vi "mp.vi"(6 "DLLPath":path, 7 "Draw":enum16{"I(Ewe)", "Ewe(t)", "I(t)", "Test"}(ring)=enum."Ewe(t)", 8 "error in (no error)":errorcluster, 9 "MP Parameters":T3={"tb"=5e-05, "Scans"=[{"Value_step"=0.1, "Duration_step"=0.1, " vs_initial "=FALSE, "Record_every_dT"=0.01, "Record_every_dM"=0.01, "Mode_step"=0}, {"Value_step"=-0.2, "Duration_step"=0.1, " vs_initial "=FALSE, "Record_every_dT"=0.01, "Record_every_dM"=0.01, "Mode_step"=0}, {"Value_step"=0.0, "Duration_step"=0.1, " vs_initial "=FALSE, "Record_every_dT"=0.01, "Record_every_dM"=0.01, "Mode_step"=0}], "I_Range"=12, "Bandwidth"=5, "N_Cycles"=0, "Record_every_rc"=2, "ce"=0, "em"=1, "Step_number"=0} {"Step_number" min=0 max=1000000; "ce" items=["Standard", "CE to ground"]; "N_Cycles" min=0 max=1000000; "Bandwidth" items=["1"=1, "2"=2, "3"=3, "4"=4, "5"=5, "6"=6, "7"=7, "8"=8, "9"=9]; "I_Range" items=["1pA", "1nA", "10nA", "100nA", "1µA", "10µA", "100µA", "1mA", "10mA", "100mA", "1A", "Booster", "Auto"]; "tb" min=5e-05 max=1 format="%^_3e"; "Scans"."Mode_step" min=0 max=1000000; "Scans"."Record_every_dM" format="%^_3e"; "Scans"."Record_every_dT" format="%^_3e"; "Scans"."Duration_step" min=1e-05 max=10 format="%^_3e"; "Scans"."Value_step" format="%^_3e"}, 10 "Channel":u8(ring) items=["1", "2", "3", "4", "5", "6", "7", "8", "9", "10", "11", "12", "13", "14", "15", "16"], 11 "IP adress":string="192.109.209.229") -> (0 "error out":errorcluster, 1 "XY Graph":cluster{"Data 101":sgl[], "Data 101":sgl[]}(graph)={"Data 101"=[8e-05, 0.1006, 0.20111999, 0.30164, 0.40219998, 0.50272, 0.60324, 0.70375997, 0.80428, 0.90484, 1.002, 1.10252, 1.20304, 1.30356, 1.40412, 1.50464, 1.60516, 1.70568, 1.8061999, 1.90676, 2.0072799, 2.1078, 2.20832, 2.3088799, 2.4094, 2.50992, 2.61044, 2.711, 2.8115199, 2.91204, 3.01256, 3.1131198, 3.21364, 3.3141599, 3.41468, 3.5152, 3.6157598, 3.71628, 3.8167999, 3.91732, 4.00108, 4.1015997, 4.20212, 4.30264, 4.4031997, 4.50372, 4.60424, 4.70476, 4.8052797, 4.90584, 5.00636, 5.1068797, 5.2074, 5.30796, 5.4084797, 5.509, 5.60952, 5.7100797, 5.8106, 5.91112], "Data 101"=[4.2835555e-07, 2.1494968e-06, 4.146294e-06, 6.138965e-06, 8.133681e-06, 1.0123058e-05, 1.2087297e-05, 1.4083101e-05, 1.6065378e-05, 1.80591e-05, 1.9984154e-05, 1.7937375e-05, 1.595267e-05, 1.3964497e-05, 1.197563e-05, 9.982255e-06, 7.9902675e-06, 6.0027883e-06, 3.9787647e-06, 1.9855738e-06, -3.2822256e-09, -1.9828094e-06, -3.9722895e-06, -5.9632257e-06, -7.95541e-06, -9.9489125e-06, -1.1902557e-05, -1.389385e-05, -1.5878555e-05, -1.7874703e-05, -1.9867039e-05, -2.1852784e-05, -2.3842693e-05, -2.583641e-05, -2.7823196e-05, -2.9813451e-05, -3.180405e-05, -3.3791526e-05, -3.5780395e-05, -3.777169e-05, -3.9435956e-05, -3.7391255e-05, -3.539476e-05, -3.3405893e-05, -3.1415642e-05, -2.9424347e-05, -2.7433402e-05, -2.5453895e-05, -2.3455323e-05, -2.1465068e-05, -1.9473428e-05, -1.7484906e-05, -1.5494306e-05, -1.3505094e-05, -1.1516228e-05, -9.523894e-06, -7.5357216e-06, -5.542347e-06, -3.5301439e-06, -1.543508e-06]}, 2 "test_output":T1, 3 "Exit 2":bool=TRUE)   [LabVIEW 2022 SP3]
doc: "The VSCAN ( Potentiodynamic Technique) consists of scanning linearly the potential of a stationary working electrode with different scan rates.\nIn general, in this VI, the first thing to do is to start by establishing the connection with the instrument defined by its IP adress, then load the firmware in the channel selected, get the information on the plugged channels, load protocol on a channel, start/stop the protocol, retreive data and draw the graph."
uses:
  Library/EClib Functions/MPParameters.ctl
  Library/EClib Functions/Parameters.ctl
  Library/EClib Functions/EClib functions.lvlib
panel:
  out "mp_data":T2
  in  "Display Parameters?":bool caption="Display Parameters"
  out "DllPath":path caption="DLL Path"
  out "LibVersion":string caption="DLL Version"
  out "Device Code":i32=12
  out "Number of points":i32=60
  out "Data 124":sgl[][](array[numeric])=[[8e-05, -0.00015008324, 4.2835555e-07, 0.0013634439, 1.0], [0.1006, 0.009902848, 2.1494968e-06, 0.010471455, 1.0], [0.20111999, 0.019955778, 4.146294e-06, 0.02059764, 1.0], [0.30164, 0.030008709, 6.138965e-06, 0.030609425, 1.0], [0.40219998, 0.04006164, 8.133681e-06, 0.04071481, 1.0], [0.50272, 0.050114572, 1.0123058e-05, 0.05077513, 1.0], [0.60324, 0.060167503, 1.2087297e-05, 0.06075918, 1.0], [0.70375997, 0.07022043, 1.4083101e-05, 0.07082297, 1.0], [0.80428, 0.08027337, 1.6065378e-05, 0.080852084, 1.0], [0.90484, 0.090326294, 1.80591e-05, 0.090902, 1.0], [1.002, 0.10004413, 1.9984154e-05, 0.100629516, 1.0], [1.10252, 0.0899912, 1.7937375e-05, 0.09124173, 1.0], [1.20304, 0.07993827, 1.595267e-05, 0.08120915, 1.0], [1.30356, 0.069885336, 1.3964497e-05, 0.0711627, 1.0], [1.40412, 0.059832405, 1.197563e-05, 0.06106771, 1.0], [1.50464, 0.049779475, 9.982255e-06, 0.051007397, 1.0], [1.60516, 0.039726544, 7.9902675e-06, 0.040967878, 1.0], [1.70568, 0.029673612, 6.0027883e-06, 0.030924892, 1.0], [1.8061999, 0.019620681, 3.9787647e-06, 0.020868042, 1.0], [1.90676, 0.009567751, 1.9855738e-06, 0.010804256, 1.0], [2.0072799, -0.00048518094, -3.2822256e-09, 0.0006746042, 1.0], [2.1078, -0.010538111, -1.9828094e-06, -0.009257445, 1.0], [2.20832, -0.020591041, -3.9722895e-06, -0.019307364, 1.0], [2.3088799, -0.030643972, -5.9632257e-06, -0.029412746, 1.0], [2.4094, -0.0406969, -7.95541e-06, -0.039452266, 1.0], [2.50992, -0.050749835, -9.9489125e-06, -0.049533386, 1.0], [2.61044, -0.060802765, -1.1902557e-05, -0.059479296, 1.0], [2.711, -0.07085569, -1.389385e-05, -0.06955695, 1.0], [2.8115199, -0.08090863, -1.5878555e-05, -0.07963461, 1.0], [2.91204, -0.09096155, -1.7874703e-05, -0.08969492, 1.0], [3.01256, -0.10101449, -1.9867039e-05, -0.09973444, 1.0], [3.1131198, -0.111067414, -2.1852784e-05, -0.1098225, 1.0], [3.21364, -0.12112035, -2.3842693e-05, -0.119851604, 1.0], [3.3141599, -0.13117327, -2.583641e-05, -0.12988071, 1.0], [3.41468, -0.1412262, -2.7823196e-05, -0.13995838, 1.0], [3.5152, -0.15127914, -2.9813451e-05, -0.15000136, 1.0], [3.6157598, -0.16133207, -3.180405e-05, -0.16006514, 1.0], [3.71628, -0.17138499, -3.3791526e-05, -0.1701324, 1.0], [3.8167999, -0.18143792, -3.5780395e-05, -0.18019964, 1.0], [3.91732, -0.19149086, -3.777169e-05, -0.19023915, 1.0], [4.00108, -0.1998683, -3.9435956e-05, -0.19861813, 1.0], [4.1015997, -0.18981537, -3.7391255e-05, -0.1892373, 1.0], [4.20212, -0.17976244, -3.539476e-05, -0.17914924, 1.0], [4.30264, -0.1697095, -3.3405893e-05, -0.16911319, 1.0], [4.4031997, -0.15965658, -3.1415642e-05, -0.15908061, 1.0], [4.50372, -0.14960365, -2.9424347e-05, -0.14899254, 1.0], [4.60424, -0.13955072, -2.7433402e-05, -0.13895303, 1.0], [4.70476, -0.12949778, -2.5453895e-05, -0.12891698, 1.0], [4.8052797, -0.119444855, -2.3455323e-05, -0.11883587, 1.0], [4.90584, -0.10939193, -2.1465068e-05, -0.10876862, 1.0], [5.00636, -0.09933899, -1.9473428e-05, -0.098690964, 1.0], [5.1068797, -0.08928607, -1.7484906e-05, -0.088686116, 1.0], [5.2074, -0.07923313, -1.5494306e-05, -0.07859806, 1.0], [5.30796, -0.069180205, -1.3505094e-05, -0.06854121, 1.0], [5.4084797, -0.059127275, -1.1516228e-05, -0.05848783, 1.0], [5.509, -0.049074344, -9.523894e-06, -0.048455246, 1.0], [5.60952, -0.039021414, -7.5357216e-06, -0.038367193, 1.0], [5.7100797, -0.028968483, -5.542347e-06, -0.028327677, 1.0], [5.8106, -0.018915553, -3.5301439e-06, -0.018236158, 1.0], [5.91112, -0.008862623, -1.543508e-06, -0.008182773, 1.0]] format="%.2f"
  in  "stop":bool
  in  "Exit":bool
  in  "Start":bool
  # "Instructions:\nBefore running the VI you must type a valid IP adress that corresponds to the instrument.Then press the Run button to execute this VI.\nWhile this VI is running, choose the available channel, enter the MP parameters or keep the default values, then press the button start to begin the experience.\nChoose the waveform to draw (Ewe(t) or I(t) or I(Ewe) or Ec(t). You can stop the measure if you press the stop button and exit the execution if you press the exit button."
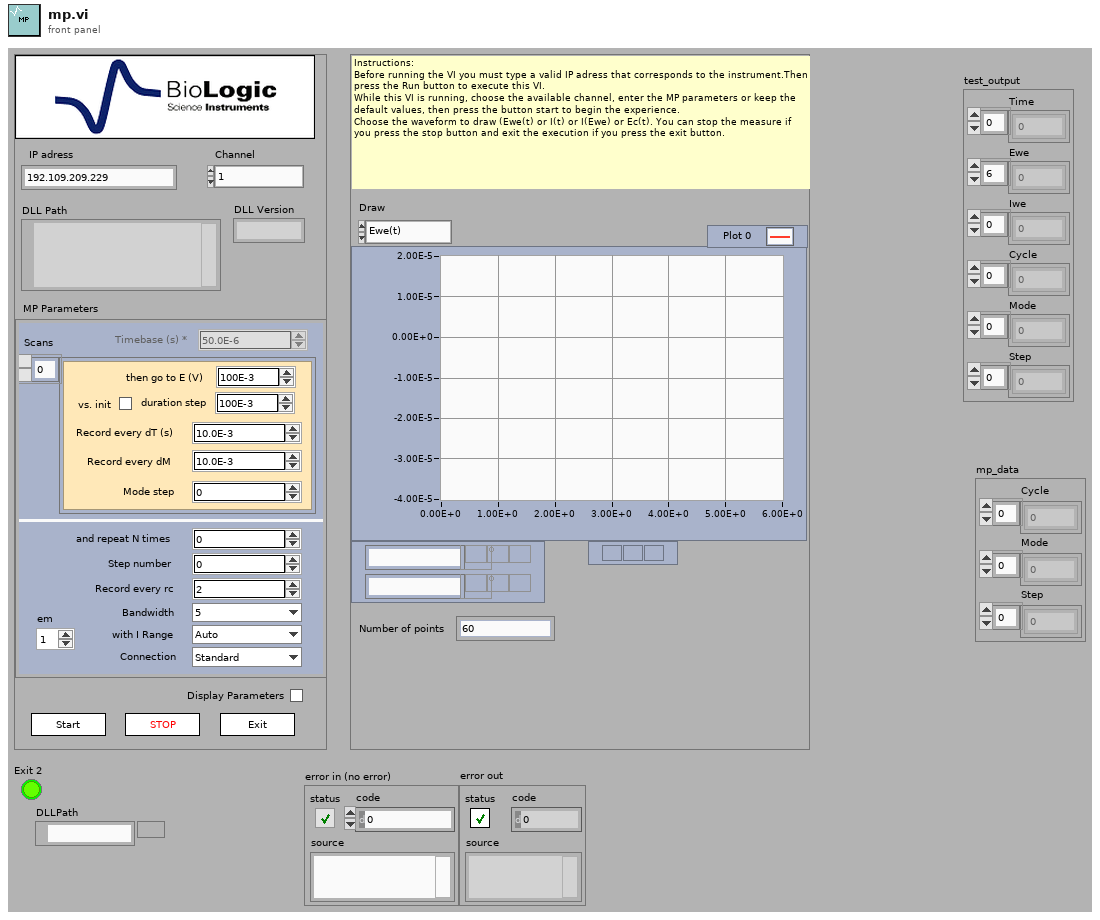
[diagram p1: front panel]
types:
  T1 = cluster{"Time":sgl[], "Ewe":sgl[], "Iwe":sgl[], "Cycle":u32[], "Mode":u32[], "Step":u32[]}
  T2 = cluster{"Cycle":u32[], "Mode":u32[], "Step":u32[]}
  T3 = typedef "EClib functions.lvlib/MPParameters.ctl" = cluster{"tb":sgl, "Scans":cluster{"Value_step":sgl, "Duration_step":sgl, " vs_initial ":bool, "Record_every_dT":sgl, "Record_every_dM":sgl, "Mode_step":i32}[], "I_Range":u16, "Bandwidth":u16, "N_Cycles":i32, "Record_every_rc":i32, "ce":u16, "em":u16, "Step_number":i32}
  T4 = cluster{"LibVersion":string, "StringLength":u32, "DllPath":path}
  T5 = cluster{"Channel":i32, "BoardVersion":i32, "BoardSerialCode":i32, "FirmwareCode":i32, "FirmwareVersion":i32, "XilinxVersion":i32, "AmpCode":i32, "NbAmp":i32, "LcBoard":i32, "Zboard":i32, "MuxBoard":i32, "GPRAboard":i32, "MemSize":i32, "MemFilled":i32, "state":i32, "MaxIRange":i32, "MinIRange":i32, "MaxBandwidth":i32, "NbOfTechniques":i32}
  T6 = typedef "EClib functions.lvlib/Parameters.ctl" = enum16{"CA", "CASG", "CP", "GEIS", "ISCAN", "OCV", "PEIS", "SCCX", "SGEIS", "SPEIS", "VSCAN", "MP"}
  T7 = typedef "EClib functions.lvlib/TechniqueParameters.ctl" = cluster{"String Label":string, "Type":i32, "Valeur":i32, "Index":i32}
  T8 = cluster{"string before end tag":string, i32, i32, i32}[]
  T9 = cluster{"IRQskipped":i32, "NbRaws":i32, "NbCols":i32, "Technique Index":i32, "TechniqueID":i32, "PrcessIndex":i32, "loop":i32, "StartTime":dbl, "MuxPad":i32}
  T10 = cluster{"State":i32, "MemFilled":i32, "TimeBase":sgl, " Ewe":sgl, " EweRangeMin":sgl, " EweRangeMax":sgl, "Ece":sgl, "EceRangeMin":sgl, "EceRangeMax":sgl, "Eoverflow":i32, "I":sgl, "IRange":i32, "Ioverflow":i32, "ElapsedTime":sgl, "Freq":sgl, "Rcomp":sgl, "Saturation":sgl, "OptErr":i32, "OptPos":i32}
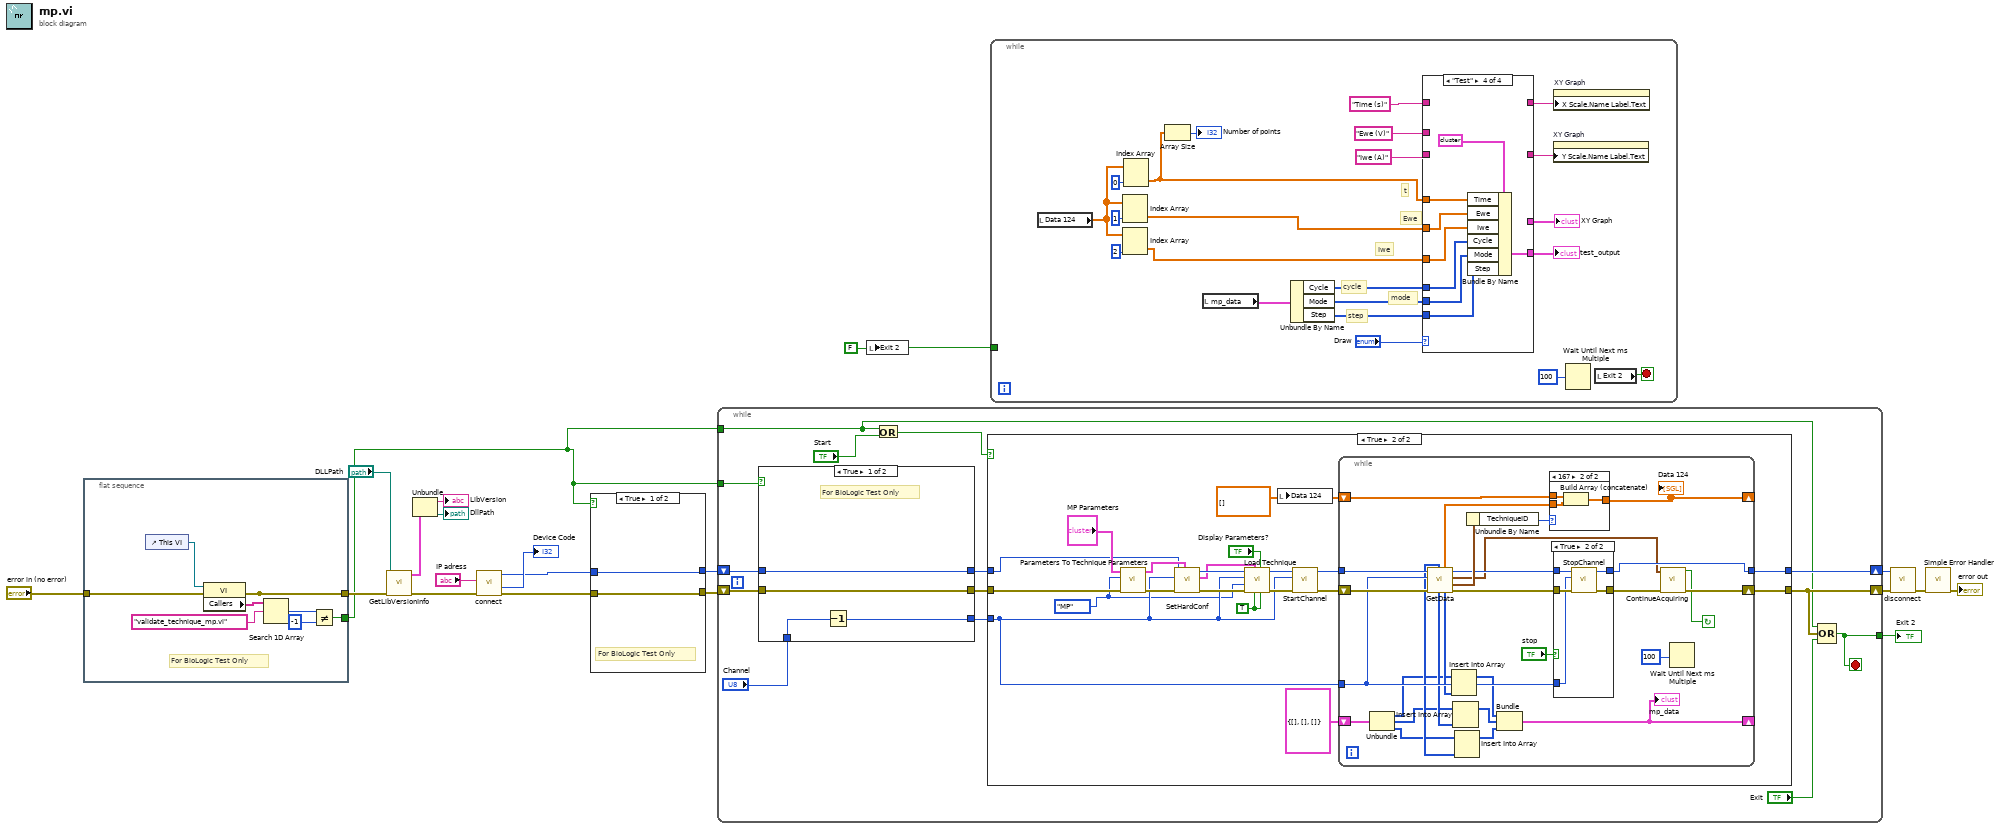
[diagram p0: block diagram]
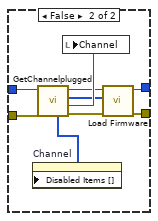
[diagram p2: hidden frame]
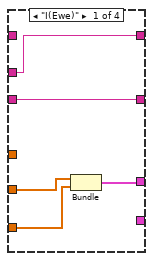
[diagram p3: hidden frame]
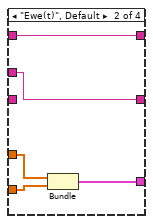
[diagram p4: hidden frame]
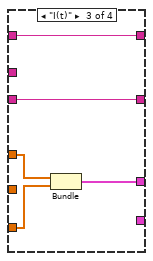
[diagram p5: hidden frame]
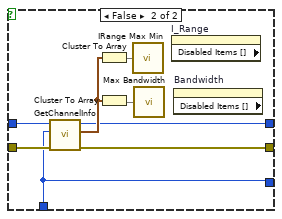
[diagram p6: hidden frame]
diagram:
  w19 = FALSE ("Exit 2")
  n1 = flat-sequence {
    tunnel: "error in (no error)" -> [w27]
    tunnel: [w21] -> _
    tunnel: [w22] -> w3
    tunnel: [w21] -> w5
    frame #0 {
      # "For BioLogic Test Only"
      n2 = control-ref of="This VI"() -> (w28:refnum<vi>)
      n3 = property class="VI"(reference=w28, error in=w27) -> (error out=w21:errorcluster, "Callers"=w26:string[])  [unwired: 1 out]
      n4 = Search 1D Array(1D array=w26, element="validate_technique_mp.vi") -> (index of element=w24:i32)  [unwired: 1 in]
      n5 = Not Equal?(x=w24, y=-1) -> (x != y?=w22:bool)
    }
  }
  n6 = call "GetLibVersionInfo.vi"("error in (no error)"=w5, "DLLPath"="DLLPath") -> ("error out"=w9:errorcluster, "LibInfo"=w12:T4)  [unwired: 8 in]
  n7 = Unbundle(w12) -> ("LibVersion"=→"LibVersion":string, "DllPath"=→"DllPath":path)  [unwired: 1 out]
  n8 = call "connect.vi"("error in (no error)"=w9, "IP"="IP adress") -> ("error out"=w16:errorcluster, "Device Code"=→"Device Code":i32, "ID Out"=w7:i32)  [unwired: 5 in, 2 out]
  n9 = case shown="True" w3 {
    tunnel: w16 -> [w30 w37]
    tunnel: [w30 w33] -> w15
    tunnel: [w29 w31] -> w6
    tunnel: w7 -> [w29 w32]
    frame True {
      # "For BioLogic Test Only"
    }
    frame False {
      n10 = call "GetChannelplugged.vi"("error in (no error)"=w37, "ID In"=w32) -> ("error out"=w36:errorcluster, "FirstPluggedChannel"=w38:u8, "PluggedChannels"=w34:u8[], "DisabledChannels"=w35:i32[])  [unwired: 5 in, 1 out]
      n11 = property on="Channel" class="Ring (strict)"("Disabled Items []"=w35) -> ()  [unwired: 2 in, 2 out]
      n12 = local write "Channel"(w38) -> ()
      n13 = call "Load Firmware.vi"("error in (no error)"=w36, "Channels"=w34, "ID In"=w32) -> ("error out"=w33:errorcluster, "ID Out"=w31:i32)  [unwired: 6 in, 1 out]
    }
  }
  n14 = while {
    shift-right: [w46] -> w14
    shift-left: w15 -> [w50]
    tunnel: [w44] -> w20
    shift-right: [w47] -> w17
    shift-left: w6 -> [w51]
    tunnel: w3 -> [w41]
    tunnel: w3 -> [w39]
    stop <- w44 stop-if-true
    n15 = case shown="True" w41 {
      tunnel: w51 -> [w54 w62]
      tunnel: w50 -> [w53 w61]
      tunnel: [w53 w60] -> w49
      tunnel: "Channel" -> [w56 w57]
      tunnel: [w54 w58] -> w48
      tunnel: [w55 w57] -> w42
      frame True {
        # "For BioLogic Test Only"
        n16 = Decrement(x=w56) -> (x-1=w55:u8)
      }
      frame False {
        n17 = call "GetChannelInfo.vi"("error in (no error)"=w61, "Channel"=w57, "ID"=w62) -> ("error out"=w60:errorcluster, "Channel information"=w59:T5, "ID Out"=w58:i32)  [unwired: 6 in]
        n18 = Cluster To Array(cluster=w59) -> (array=w64:i32[])
        n19 = Cluster To Array(cluster=w59) -> (array=w63:i32[])
        n20 = call "IRange Max Min.vi"("resources"=w64) -> ()  [unwired: 1 out]
        n21 = call "Max Bandwidth.vi"("resources"=w63) -> ()  [unwired: 1 out]
        n22 = property on="I_Range" class="Ring (strict)" props=["Disabled Items []"]() -> ()  [unwired: 2 in, 3 out]
        n23 = property on="Bandwidth" class="Ring (strict)" props=["Disabled Items []"]() -> ()  [unwired: 2 in, 3 out]
      }
    }
    n24 = Or(x=w39, y="Start") -> (x .or. y?=w40:bool)
    n25 = case shown="True" w40 {
      tunnel: w42 -> [_ w69]
      tunnel: [w66 w80] -> w46
      tunnel: w49 -> [w66 w72]
      tunnel: w48 -> [w65 w68]
      tunnel: [w65 w79] -> w47
      frame False {
      }
      frame True {
        w67 = Parameters."MP" ("Parameters")
        w85 = TRUE ("First Protocol")
        w86 = sgl[][] []
        n26 = call "Parameters To Technique Parameters.vi"("error in (no error)"=w72, "Parameters"=w67, "ParameterIN"="MP Parameters") -> ("error out"=w78:errorcluster, "Params Values"=w74:T7[])  [unwired: 7 in]
        n27 = call "SetHardConf.vi"("Params Values"=w74, "error in (no error)"=w78, "Channel"=w69, "ID In"=w68) -> ("error out"=w77:errorcluster, "Params Values Trimed"=w75:T8, "ID Out"=w76:i32)  [unwired: 5 in]
        n28 = call "Load Technique.vi"("Last Protocol"=w85, "Display Parameters?"="Display Parameters?", "First Protocol"=w85, "TechniqueParameters"=w75, "error in (no error)"=w77, "Parameters"=w67, "Selected Channel"=w69, "ID In"=w76) -> ("error out"=w84:errorcluster, "ID  Out"=w83:i32)  [unwired: 1 in, 1 out]
        n29 = local write "Data 124"(w86) -> ()
        n30 = call "StartChannel.vi"("error in (no error)"=w84, "Channel"=w69, "ID In"=w83) -> ("error out"=w82:errorcluster, "ID Out"=w81:i32)  [unwired: 7 in]
        n31 = while {
          shift-right: [w101] -> w80
          shift-left: w82 -> [w113]
          shift-right: [w110] -> _
          shift-left: w86 -> [w111]
          tunnel: w69 -> [w103]
          tunnel: w81 -> [w105]
          tunnel: [w102] -> w79
          shift-right: [w91] -> _
          shift-left: cluster{u32[], u32[], u32[]} {[], [], []} -> [w90]
          stop <- w99 continue-if-true
          n32 = Unbundle(w90) -> (w89:u32[], w87:u32[], w88:u32[])
          n33 = call "GetData.vi"("error in (no error)"=w113, "Channel"=w103, "ID In"=w105) -> ("error out"=w109:errorcluster, "Data information"=w114:T9, "Current values"=w98:T10, "ID Out"=w104:i32, "row2"=w97:u32[], "Data"=w106:dbl[][], "row3"=w96:u32[], "row4"=w95:u32[])  [unwired: 1 in]
          n34 = Insert Into Array(array=w89, new element=w97) -> (w94:u32[])  [unwired: 1 in]
          n35 = Insert Into Array(array=w87, new element=w96) -> (w93:u32[])  [unwired: 1 in]
          n36 = Insert Into Array(array=w88, new element=w95) -> (w92:u32[])  [unwired: 1 in]
          n37 = Unbundle By Name(w114) -> ("TechniqueID"=w108:i32)
          n38 = Bundle(w94, w93, w92) -> (w91:cluster{u32[], u32[], u32[]})  [unwired: 1 in]
          "mp_data" <- w91
          n39 = case shown="167" w108 {
            tunnel: w106 -> [_ w125]
            tunnel: w111 -> [w122 w124]
            tunnel: [w122 w123] -> w110
            frame 0, Default {
            }
            frame 167 {
              n40 = Build Array (concatenate)(w124, w125) -> (w123:dbl[][])
            }
          }
          "Data 124" <- w110
          n41 = case shown="True" "stop" {
            tunnel: [w116 w121] -> w100
            tunnel: w109 -> [w116 w120]
            tunnel: w104 -> [w115 w119]
            tunnel: w103 -> [_ w118]
            tunnel: [w115 w117] -> w102
            frame False {
            }
            frame True {
              n42 = call "StopChannel.vi"("error in (no error)"=w120, "Channel"=w118, "ID In"=w119) -> ("error out"=w121:errorcluster, "ID Out"=w117:i32)  [unwired: 7 in]
            }
          }
          n43 = call "ContinueAcquiring.vi"("error in"=w100, "Current values"=w98) -> ("error out"=w101:errorcluster, "ContinueAcquiring?"=w99:bool)  [unwired: 8 in]
          n44 = Wait Until Next ms Multiple(millisecond multiple=u32 100) -> ()  [unwired: 1 out]
        }
      }
    }
    n45 = Compound Arithmetic op=OR(w39, w46, "Exit") -> (w44:bool)
  }
  "Exit 2" <- w20
  n46 = local write "Exit 2"(w19) -> ()
  n47 = while {
    tunnel: w19 -> [_]
    stop <- w146 stop-if-true
    # "step"
    # "mode"
    # "cycle"
    # "Ewe"
    # "Iwe"
    # "t"
    n48 = local read "Data 124"() -> (w131:sgl[][])
    n49 = Index Array(array=w131, index (col)=1 ("Index")) -> (element=w133:sgl[])  [unwired: 1 in]
    n50 = Index Array(array=w131, index (col)=2 ("Index")) -> (element=w132:sgl[])  [unwired: 1 in]
    n51 = Index Array(array=w131, index (col)=0 ("Index")) -> (element=w134:sgl[])  [unwired: 1 in]
    n52 = Array Size(array=w134) -> (size(s)=→"Number of points":i32)
    n53 = local read "mp_data"() -> (w130:T2)
    n54 = Unbundle By Name(w130) -> ("Cycle"=w129:u32[], "Mode"=w128:u32[], "Step"=w127:u32[])
    n55 = case shown="\"Test\"" "Draw" {
      tunnel: w134 -> [_ w157 w162 w167]
      tunnel: w132 -> [w150 _ w161 w166]
      tunnel: [w149 w154 w158 _] -> w141
      tunnel: "Ewe (V)" ("Y Scale.Name Label.Text") -> [w152 w156 _ _]
      tunnel: "Iwe (A)" ("Y Scale.Name Label.Text") -> [w151 _ w160 _]
      tunnel: [w151 w156 w160 _] -> w140
      tunnel: [w152 w155 w159 _] -> w139
      tunnel: "Time (s)" ("Y Scale.Name Label.Text") -> [_ w155 w159 _]
      tunnel: w129 -> [_ _ _ w169]
      tunnel: w133 -> [w148 w153 _ w168]
      tunnel: [_ _ _ w170] -> w126
      tunnel: w128 -> [_ _ _ w165]
      tunnel: w127 -> [_ _ _ w164]
      frame "I(Ewe)" {
        n56 = Bundle("Data 124"=w148, "Data 124"=w150) -> (w149:cluster{"Data 124":sgl[], "Data 124":sgl[]})  [unwired: 1 in]
      }
      frame "Ewe(t)", Default {
        n57 = Bundle("Data 124"=w157, "Data 124"=w153) -> (w154:cluster{"Data 124":sgl[], "Data 124":sgl[]})  [unwired: 1 in]
      }
      frame "I(t)" {
        n58 = Bundle("Data 124"=w162, "Data 124"=w161) -> (w158:cluster{"Data 124":sgl[], "Data 124":sgl[]})  [unwired: 1 in]
      }
      frame "Test" {
        n59 = Bundle By Name(cluster=T1 {"Time"=[0.0, 0.0001, 0.114099994, 0.1218, 0.14999999, 0.19999999, 0.25, 0.29999998, 0.35, 0.39999998, 0.45, 0.5, 0.55, 0.59999996, 0.65, 0.7, 0.75, 0.79999995, 0.84999996, 0.9, 0.95, 1.0, 1.05, 1.1, 1.15, 1.1999999, 1.25, 1.3, 1.35, 1.4, 1.4499999, 1.5, 1.55, 1.5999999, 1.65, 1.6999999, 1.75, 1.8, 1.8499999, 1.9, 1.9499999, 2.0, 2.05, 2.1, 2.1499999, 2.2, 2.25, 2.3, 2.35, 2.3999999, 2.45, 2.5, 2.55, 2.6, 2.6499999, 2.7, 2.75, 2.8, 2.85, 2.8999999, 2.9499998, 3.0, 3.0003, 3.0009, 3.0031998, 3.0091, 3.0203, 3.0379, 3.05, 3.0793998, 3.1, 3.146, 3.1499999, 3.1999998, 3.25, 3.3, 3.35, 3.3999999, 3.4499998, 3.5, 3.55, 3.6, 3.6499999, 3.6999998, 3.75, 3.8, 3.85, 3.8999999, 3.9499998, 4.0, 4.0499997, 4.1, 4.15, 4.2, 4.25, 4.2999997, 4.35, 4.4, 4.45, 4.5, 4.5499997, 4.6, 4.65, 4.7, 4.75, 4.7999997, 4.85, 4.9, 4.95, 5.0, 5.0499997, 5.1, 5.15, 5.2, 5.25, 5.2999997, 5.35, 5.4, 5.45, 5.5, 5.5499997, 5.6, 5.65, 5.7, 5.75, 5.7999997, 5.85, 5.8999996, 5.95, 6.0], "Ewe"=[0.0, 2.0333483, 2.370001, 2.26923, 2.2448394, 2.2499743, 2.2618487, 2.2766113, 2.291053, 2.3051739, 2.3205783, 2.335341, 2.3497827, 2.3632617, 2.378987, 2.392466, 2.4072287, 2.4203868, 2.4348285, 2.4492702, 2.4630702, 2.4781537, 2.4922745, 2.5054326, 2.5192325, 2.5336742, 2.546832, 2.560632, 2.57379, 2.5882318, 2.6004272, 2.6151898, 2.6286688, 2.6411848, 2.6546638, 2.667501, 2.6822636, 2.6954217, 2.7082586, 2.7217376, 2.7348957, 2.7474117, 2.7605698, 2.7743697, 2.786886, 2.799723, 2.8115973, 2.8250763, 2.8375924, 2.8513923, 2.8623037, 2.8767457, 2.8889408, 2.9011362, 2.9126894, 2.9261684, 2.9386845, 2.9515216, 2.9630752, 2.976554, 2.9884284, 3.0006235, 1.9993299, 2.0006137, 2.0006137, 2.0012555, 2.0002928, 2.0002928, 2.0015764, 2.0002928, 2.0012555, 2.0018973, 1.9999717, 2.0012555, 2.0006137, 2.0012555, 2.0009346, 2.0012555, 2.0006137, 2.0022182, 2.0009346, 2.0006137, 2.0012555, 2.0009346, 1.9996508, 2.0006137, 2.0002928, 2.0002928, 2.0009346, 2.0012555, 1.9999717, 2.0006137, 2.0006137, 2.0015764, 2.0002928, 2.0006137, 2.0012555, 2.0012555, 2.0018973, 2.0006137, 2.0006137, 2.0012555, 2.0015764, 2.0006137, 2.0006137, 2.0022182, 2.0006137, 2.0006137, 2.0002928, 2.0006137, 2.0006137, 2.0006137, 2.0002928, 1.9996508, 2.0006137, 2.0006137, 2.0002928, 2.0002928, 1.9996508, 2.0012555, 2.0006137, 2.0012555, 2.0012555, 2.0009346, 2.0006137, 1.9999717, 2.0012555, 2.0006137, 1.9999717, 2.0009346], "Iwe"=[0.0, 9.619652e-06, 0.068132386, 0.068285085, 0.06805604, 0.06866684, 0.068437785, 0.06775063, 0.06836144, 0.06820874, 0.068285085, 0.06851414, 0.06851414, 0.06859049, 0.06874319, 0.06820874, 0.068437785, 0.06836144, 0.068437785, 0.06859049, 0.06851414, 0.06851414, 0.068437785, 0.06836144, 0.068437785, 0.067979686, 0.06836144, 0.06851414, 0.068285085, 0.06851414, 0.06805604, 0.06782699, 0.068285085, 0.068132386, 0.06820874, 0.06836144, 0.06820874, 0.06805604, 0.06836144, 0.06820874, 0.06805604, 0.06851414, 0.06874319, 0.06851414, 0.06866684, 0.06859049, 0.06866684, 0.06851414, 0.068285085, 0.06866684, 0.06851414, 0.068437785, 0.06851414, 0.067979686, 0.068285085, 0.06889589, 0.068132386, 0.06790333, 0.068285085, 0.06851414, 0.06790333, 0.06820874, -1.2395995, -1.1262953, -1.0223823, -0.92106515, -0.8207405, -0.72033954, -0.66704684, -0.56611145, -0.5096121, -0.40936384, -0.4017288, -0.3224006, -0.2617019, -0.21489905, -0.17809808, -0.14740518, -0.12579797, -0.10480158, -0.09014227, -0.07693363, -0.06708441, -0.057846002, -0.050287303, -0.04439365, -0.039257187, -0.034876317, -0.03131972, -0.028007349, -0.025160545, -0.022931946, -0.020718614, -0.018841095, -0.017375715, -0.015895072, -0.014757877, -0.013483303, -0.012552175, -0.011682106, -0.010850199, -0.010338842, -0.009453508, -0.0091863815, -0.008697922, -0.008064451, -0.0076599447, -0.007072266, -0.00698068, -0.0064311633, -0.0061106114, -0.005973232, -0.0056659016, -0.0054008486, -0.005249608, -0.004974625, -0.004819565, -0.0046209665, -0.0044223676, -0.004220713, -0.004090096, -0.003931217, -0.0038143494, -0.0036860236, -0.0035324916, -0.0034347198, -0.0033392396, -0.0032261908, -0.0031383492, -0.0030237727], "Cycle"=[0, 0, 0, 0, 0, 0, 0, 0, 0, 0, 0, 0, 0, 0, 0, 0, 0, 0, 0, 0, 0, 0, 0, 0, 0, 0, 0, 0, 0, 0, 0, 0, 0, 0, 0, 0, 0, 0, 0, 0, 0, 0, 0, 0, 0, 0, 0, 0, 0, 0, 0, 0, 0, 0, 0, 0, 0, 0, 0, 0, 0, 0, 0, 0, 0, 0, 0, 0, 0, 0, 0, 0, 0, 0, 0, 0, 0, 0, 0, 0, 0, 0, 0, 0, 0, 0, 0, 0, 0, 0, 0, 0, 0, 0, 0, 0, 0, 0, 0, 0, 0, 0, 0, 0, 0, 0, 0, 0, 0, 0, 0, 0, 0, 0, 0, 0, 0, 0, 0, 0, 0, 0, 0, 0, 0, 0, 0, 0, 0, 0], "Mode"=[0, 0, 1, 1, 1, 1, 1, 1, 1, 1, 1, 1, 1, 1, 1, 1, 1, 1, 1, 1, 1, 1, 1, 1, 1, 1, 1, 1, 1, 1, 1, 1, 1, 1, 1, 1, 1, 1, 1, 1, 1, 1, 1, 1, 1, 1, 1, 1, 1, 1, 1, 1, 1, 1, 1, 1, 1, 1, 1, 1, 1, 1, 0, 0, 0, 0, 0, 0, 0, 0, 0, 0, 0, 0, 0, 0, 0, 0, 0, 0, 0, 0, 0, 0, 0, 0, 0, 0, 0, 0, 0, 0, 0, 0, 0, 0, 0, 0, 0, 0, 0, 0, 0, 0, 0, 0, 0, 0, 0, 0, 0, 0, 0, 0, 0, 0, 0, 0, 0, 0, 0, 0, 0, 0, 0, 0, 0, 0, 0, 0], "Step"=[0, 0, 0, 0, 0, 0, 0, 0, 0, 0, 0, 0, 0, 0, 0, 0, 0, 0, 0, 0, 0, 0, 0, 0, 0, 0, 0, 0, 0, 0, 0, 0, 0, 0, 0, 0, 0, 0, 0, 0, 0, 0, 0, 0, 0, 0, 0, 0, 0, 0, 0, 0, 0, 0, 0, 0, 0, 0, 0, 0, 0, 0, 1, 1, 1, 1, 1, 1, 1, 1, 1, 1, 1, 1, 1, 1, 1, 1, 1, 1, 1, 1, 1, 1, 1, 1, 1, 1, 1, 1, 1, 1, 1, 1, 1, 1, 1, 1, 1, 1, 1, 1, 1, 1, 1, 1, 1, 1, 1, 1, 1, 1, 1, 1, 1, 1, 1, 1, 1, 1, 1, 1, 1, 1, 1, 1, 1, 1, 1, 1]} ("test_output"), "Time"=w167, "Ewe"=w168, "Iwe"=w166, "Cycle"=w169, "Mode"=w165, "Step"=w164) -> (w170:T1)
      }
    }
    "XY Graph" <- w141
    "test_output" <- w126
    n60 = property on="XY Graph" class="XYGraph (strict)"("Y Scale.Name Label.Text"=w140) -> ()  [unwired: 2 in, 2 out]
    n61 = property on="XY Graph" class="XYGraph (strict)"("X Scale.Name Label.Text"=w139) -> ()  [unwired: 2 in, 2 out]
    n62 = Wait Until Next ms Multiple(millisecond multiple=u32 100) -> ()  [unwired: 1 out]
    n63 = local read "Exit 2"() -> (w146:bool)
  }
  n64 = call "disconnect.vi"("error in (no error)"=w14, "ID In"=w17) -> ("error out"=w13:errorcluster)  [unwired: 9 in]
  n65 = call <vilib>:"Simple Error Handler.vi"("error in (no error)"=w13) -> ("error out"=→"error out":errorcluster)  [unwired: 4 in, 4 out]
